vi "subFGV.vi"(6 "CAN Data":u8[](array[numeric]), 9 "DLC (8)":u8, 10 "MSG type":enum8{"STD", "RTR", "XTD", "XTD RTR", "STATUS"}(ring), 11 "Identifier":u32) -> (3 "Chaîne":string)   [LabVIEW 2020, in "PEAK_lib_ALEX.lvlib"]
uses:
  PEAK_lib_ALEX.lvlib
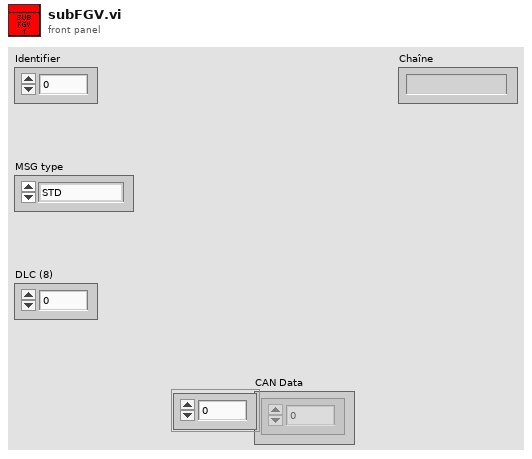
[diagram p1: front panel]
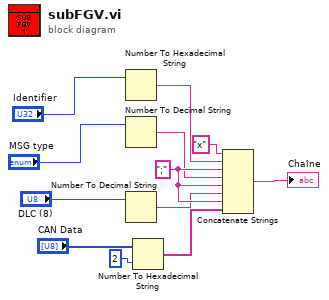
[diagram p0: block diagram]
diagram:
  w7 = ";" ("chaîne")
  n1 = Number To Hexadecimal String(2:"Identifier") -> (0:w2:string)  [unwired: 1 in]
  n2 = Number To Decimal String(number="MSG type") -> (decimal integer string=w3:string)  [unwired: 1 in]
  n3 = Number To Decimal String(number="DLC (8)") -> (decimal integer string=w6:string)  [unwired: 1 in]
  n4 = Number To Hexadecimal String(1:i16 2 ("largeur (-)"), 2:"CAN Data") -> (0:w12:string[])
  n5 = Concatenate Strings("x" ("chaîne"), w2, w7, w3, w7, w6, w7, w12) -> (→"Chaîne":string)
